vi "Send Return Microgrid State.vi"(5 "Message Type":refnum<class "Return Microgrid State Msg.lvclass">, 7 "Message Priority (Normal)":T2=enum."Normal", 8 "error in (no error)":errorcluster, 10 "Microgrid State":T1, 11 "Message Enqueuer":refnum<class "Message Enqueuer.lvclass">) -> (0 "error out":errorcluster, 3 "Message Enqueuer out":refnum<class "Message Enqueuer.lvclass">)   [LabVIEW 2018, in "EMS Core.lvlib" / "Return Microgrid State Msg.lvclass"]
doc: "This VI sends the message to an actor."
uses:
  Return Microgrid State Msg.lvclass
  <vilib>/ActorFramework/Message Enqueuer/Message Enqueuer.lvclass
  <vilib>/ActorFramework/Message Enqueuer/Message Priority.ctl
  C:/Program Files (x86)/National Instruments/LabVIEW 2018/vi.lib/ActorFramework/Message/Message.lvclass
  EMS/Controls/Microgrid State.ctl
  Return Microgrid State Msg.lvclass/Return Microgrid State Msg.ctl
  <vilib>/ActorFramework/Message Enqueuer/Message Enqueuer.lvclass/Message Enqueuer.ctl
  <vilib>/ActorFramework/Message Priority Queue/Priority Enqueue.vi
  EMS/EMS.lvclass
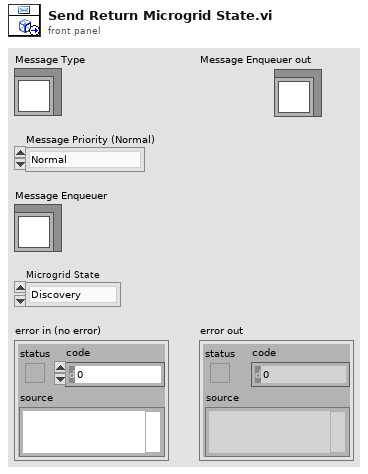
[diagram p1: front panel]
types:
  T1 = typedef "EMS Core.lvlib/EMS.lvclass/Microgrid State.ctl" = enum16{"Discovery", "Commissioning", "Activation", "Blackstart", "OnGrid", "OffGrid", "Island", "Resynchronization", "Manual", "Shutdown", "Stop"}
  T2 = typedef "Actor Framework.lvlib/Message Enqueuer.lvclass/Message Priority.ctl" = enum16{"Low", "Normal", "High"}
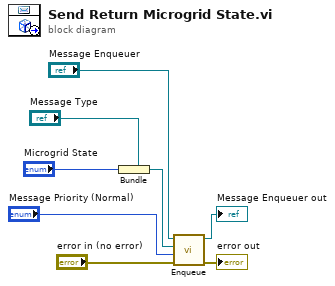
[diagram p0: block diagram]
diagram:
  n1 = Bundle(cluster="Message Type", "Microgrid State") -> (w4:refnum<class "Return Microgrid State Msg.lvclass">)
  n2 = call <vilib>:"Enqueue.vi"("error in (no error)"="error in (no error)", "Message Priority (Normal)"="Message Priority (Normal)", "Message"=w4, "Message Enqueuer in"="Message Enqueuer") -> ("error out"=→"error out":errorcluster, "Message Enqueuer out"=→"Message Enqueuer out":refnum<class "Message Enqueuer.lvclass">)  [unwired: 6 in]
